vi "SetWl.vi"(0 "VISA resource name":refnum<visa-resource-name>="COM3", 2 "Wavelength (nm)":sgl=600.001 format="%.3f", 5 "error in (no error)":errorcluster) -> (14 "VISA resource name out":refnum<visa-resource-name>, 19 "error out":errorcluster)   [LabVIEW 2016]
doc: "Function: tga1240_config_pulse\n\nPurpose: Configure the parameters for a pulse waveform"
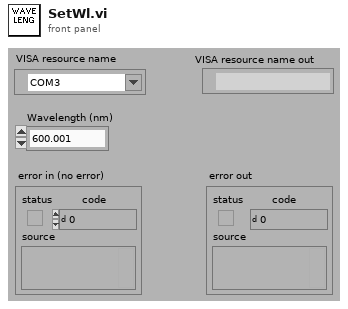
[diagram p1: front panel]
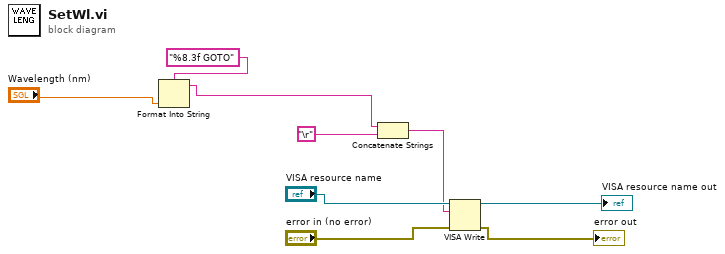
[diagram p0: block diagram]
diagram:
  n1 = Format Into String(format string="%8.3f GOTO", "Wavelength (nm)") -> (resulting string=w1:string)  [unwired: 2 in, 1 out]
  n2 = Concatenate Strings(w1, "\r") -> (w5:string)
  n3 = VISA Write(VISA resource name="VISA resource name", write buffer=w5, error in (no error)="error in (no error)") -> (VISA resource name out=→"VISA resource name out":refnum<visa-resource-name>, error out=→"error out":errorcluster)  [unwired: 1 out]
